vi "Act2_mandar.vi"() -> ()   [LabVIEW 2020]
uses:
  <vilib>/httpClient/PUTBuffer.vi
  <vilib>/httpClient/LabVIEWHTTPClient.lvlib
panel:
  out "headers 2":string
  out "body":string
  out "error out 2":errorcluster
  in  "Temperatura":dbl(slide) scale=0.0..100.0
  in  "Lateral":bool
  in  "Frontal":bool
  out "headers":string
  in  "stop":bool
  out "error out":errorcluster
  out "body4":string
  in  "Humedad":dbl(knob) scale=0.0..10.0
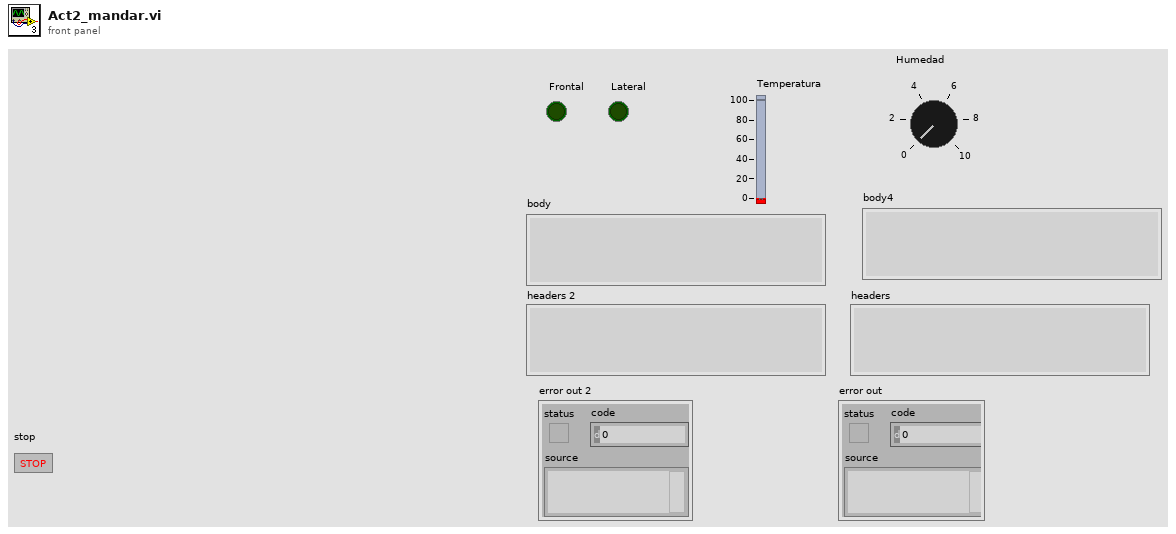
[diagram p1: front panel]
types:
  T1 = cluster{"Frontal":bool, "Lateral":bool, "Temperatura":dbl}
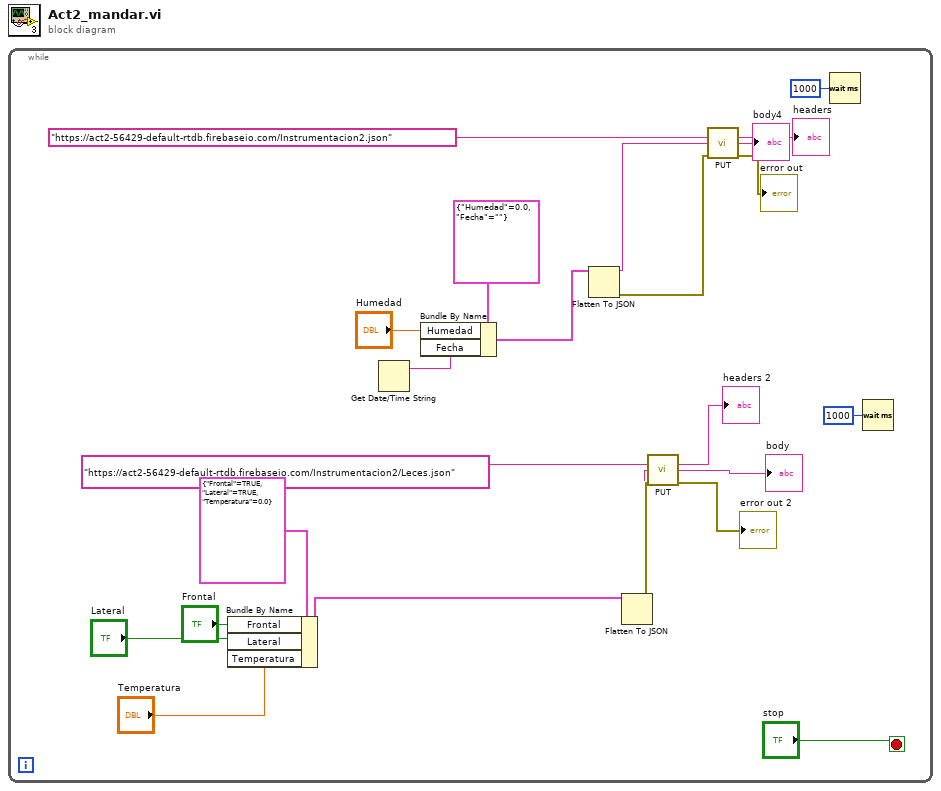
[diagram p0: block diagram]
diagram:
  n1 = while {
    stop <- "stop" stop-if-true
    n2 = Bundle By Name(cluster=T1 {"Frontal"=TRUE, "Lateral"=TRUE, "Temperatura"=0.0}, "Frontal"="Frontal", "Lateral"="Lateral", "Temperatura"="Temperatura") -> (w7:T1)
    n3 = Get Date/Time String() -> (date string=w1:string)  [unwired: 3 in, 1 out]
    n4 = Bundle By Name(cluster=cluster{"Humedad":dbl, "Fecha":string} {"Humedad"=0.0, "Fecha"=""}, "Humedad"="Humedad", "Fecha"=w1) -> (w18:cluster{"Humedad":dbl, "Fecha":string})
    n5 = Flatten To JSON(anything=w18) -> (JSON string=w17:string, 11:w16:errorcluster)  [unwired: 2 in]
    n6 = Flatten To JSON(anything=w7) -> (JSON string=w5:string, 11:w6:errorcluster)  [unwired: 2 in]
    n7 = call-poly <vilib>:"PUT.vi"("url"="https://act2-56429-default-rtdb.firebaseio.com/Instrumentacion2/Leces.json" ("string"), "buffer"=w5, "error in (no error)"=w6) -> ("headers"=→"headers 2":string, "body"=→"body":string, "error out"=→"error out 2":errorcluster)  [unwired: 9 in, 1 out]
    n8 = call-poly <vilib>:"PUT.vi"("url"="https://act2-56429-default-rtdb.firebaseio.com/Instrumentacion2.json" ("string"), "buffer"=w17, "error in (no error)"=w16) -> ("headers"=→"headers":string, "body"=→"body4":string, "error out"=→"error out":errorcluster)  [unwired: 9 in, 1 out]
    n9 = Wait (ms)(milliseconds to wait=u32 1000) -> ()  [unwired: 1 out]
    n10 = Wait (ms)(milliseconds to wait=u32 1000) -> ()  [unwired: 1 out]
  }
